vi "QZ Decomposition.vi"   [LabVIEW 2020, in "NI_AALPro.lvlib"]
doc: "Performs the QZ decomposition of a pair of square matrices. The data types you wire to the <B>A</B> and <B>B</B> inputs determine the polymorphic instance to use."
uses:
  <vilib>/Analysis/NI_AALPro.lvlib
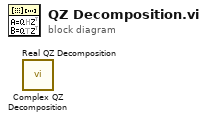
[diagram p0: block diagram]
diagram:
  n1 = call <vilib>:"Complex QZ Decomposition.vi"() -> ()  [unwired: 10 in, 6 out]
  n2 = call <vilib>:"Real QZ Decomposition.vi"() -> ()  [unwired: 10 in, 6 out]
